vi "visionCalc.vi"(0 "imgWidth":dbl, 2 "leftX":dbl, 3 "rightX":dbl) -> (7 "angle (deg)":dbl, 10 "distance (ft)":dbl)   [LabVIEW 2016]
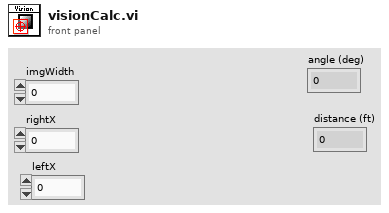
[diagram p1: front panel]
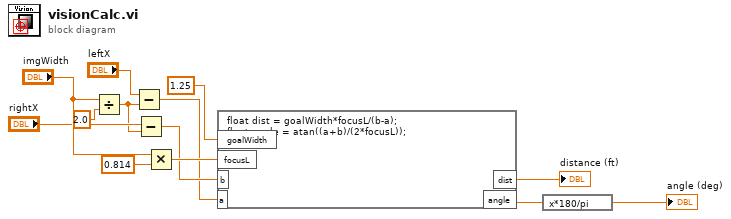
[diagram p0: block diagram]
diagram:
  n1 = Divide(x="imgWidth", y=2.0) -> (x/y=w4:dbl)
  n2 = Subtract(x="leftX", y=w4) -> (x-y=w6:dbl)
  n3 = Subtract(x="rightX", y=w4) -> (x-y=w7:dbl)
  n4 = Multiply(x="imgWidth", y=0.814) -> (x*y=w12:dbl)
  n5 = formula code="float dist = goalWidth*focusL/(b-a);\nfloat angle = atan((a+b)/(2*focusL));"("goalWidth"=1.25 ("input variable"), "focusL"=w12, "b"=w7, "a"=w6) -> ("dist"=→"distance (ft)":dbl, "angle"=w13:dbl)
  n6 = expression code="x*180/pi"(w13) -> (→"angle (deg)":dbl)
